vi "Initialize gain.vi"(7 "Status":T1 {"Setting"."X Pos." scale=-2.0..2.0; "Setting"."Y Pos." scale=-2.0..2.0}, 10 "错误输入（无错误）":errorcluster, 11 "Event Controls":T4 {"Gain" scale=0.0..150.0}) -> (2 "error out":errorcluster)   [LabVIEW 2013]
uses:
  GUI control.ctl
  init & communication/init-status.ctl
  init & communication/Setting.ctl
  init & communication/event-package.ctl
  init & communication/Event1.ctl
  init & communication/data-package.ctl
  init & communication/Event.ctl
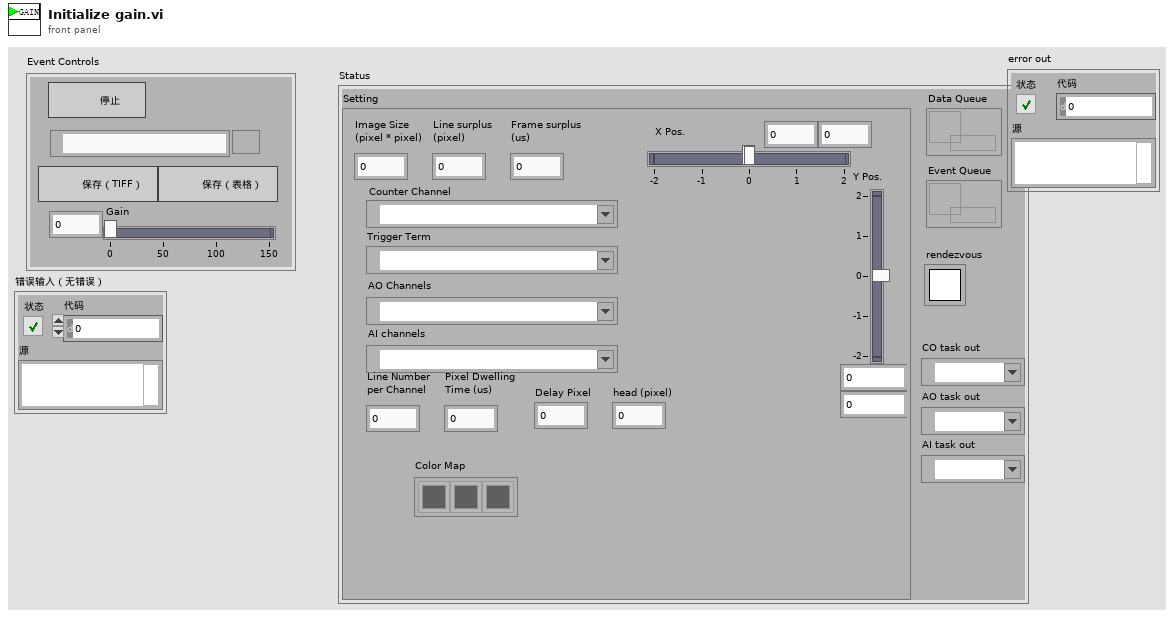
[diagram p1: front panel]
types:
  T1 = typedef "init-status.ctl" = cluster{"Setting":T2, "Event Queue":refnum<queue>, "Data Queue":refnum<queue>, "rendezvous":T3, "CO task out":refnum<k21>, "AO task out":refnum<k21>, "AI task out":refnum<k21>}
  T2 = typedef "Setting.ctl" = cluster{"Image Size\n(pixel * pixel)":i32, "Counter Channel":tag, "Trigger Term":tag, "AO Channels":tag, "Y Pos.":cluster{dbl, dbl}, "X Pos.":cluster{dbl, dbl}, "Line surplus\n(pixel)":i32, "Frame surplus\n(us)":i32, "AI channels":tag, "Line Number\nper Channel":i32, "Delay Pixel":i32, "Pixel Dwelling\nTime (us)":i32, "Color Map":u32[], "head (pixel)":i32}
  T3 = typedef "Rendezvous RefNum" = refnum<k1>
  T4 = typedef "GUI control.ctl" = cluster{"stop":bool, "save sheet":bool, "Path":path, "save tiff":bool, "Gain":dbl}
  T5 = typedef "event-package.ctl" = cluster{"Event":T6, "Data":string}
  T6 = typedef "Event1.ctl" = enum16{"null", "stop AI", "stop AO", "stop Imaging", "stop Counter", "save sheet", "restart", "save tiff", "gain changed"}
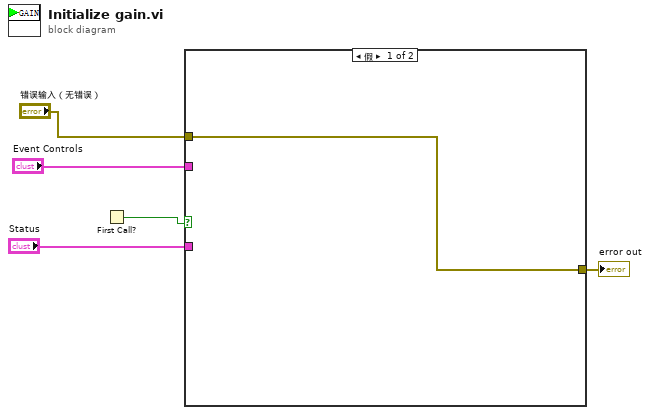
[diagram p0: block diagram]
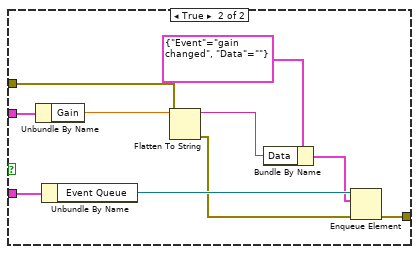
[diagram p2: hidden frame]
diagram:
  n1 = First Call?() -> (First Call?: T/F=w5:bool)
  n2 = case shown="假" w5 {
    tunnel: "Event Controls" -> [_ w14]
    tunnel: "Status" -> [_ w16]
    tunnel: "错误输入（无错误）" -> [w6 w8]
    tunnel: [w6 w7] -> w1
    frame False {
    }
    frame True {
      n3 = Unbundle By Name(w14) -> ("Gain"=w13:dbl)
      n4 = Unbundle By Name(w16) -> ("Event Queue"=w15:refnum<queue>)
      n5 = Flatten To String(anything=w13, error in (no error)=w8) -> (data string=w10:string, error out=w9:errorcluster)  [unwired: 2 in, 1 out]
      n6 = Bundle By Name(cluster=T5 {"Event"=enum."gain changed", "Data"=""} ("元素"), "Data"=w10) -> (w11:T5)
      n7 = Enqueue Element(queue=w15, element=w11, error in (no error)=w9) -> (error out=w7:errorcluster)  [unwired: 1 in, 2 out]
    }
  }
  "error out" <- w1
